vi "Close.vi"(8 "error in (no error)":errorcluster, 11 "FgenPluginsBase in":refnum<class "FgenPluginsBase.lvclass">) -> (0 "error out":errorcluster, 3 "FgenPluginsBase out":refnum<class "FgenPluginsBase.lvclass">)   [LabVIEW 2014, in "FgenPlugins.lvlib" / "FgenPluginsBase.lvclass"]
uses:
  FgenPluginsBase.lvclass
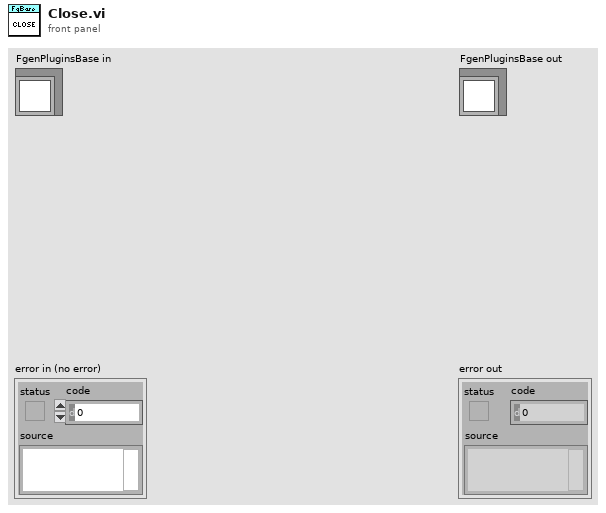
[diagram p1: front panel]
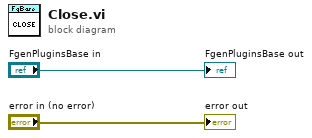
[diagram p0: block diagram]
diagram:
  "error out" <- "error in (no error)"
  "FgenPluginsBase out" <- "FgenPluginsBase in"
